vi "Is OceanOptics installed.vi"(8 "Error In":errorcluster) -> (0 "Error Out":errorcluster, 3 "file or folder exists?":bool)   [LabVIEW 2016]
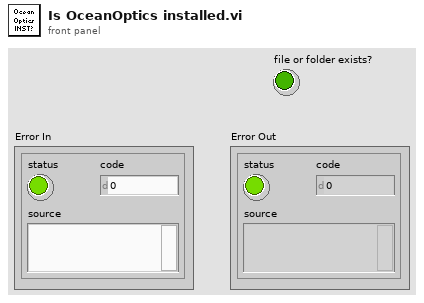
[diagram p1: front panel]
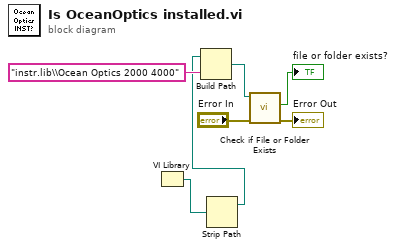
[diagram p0: block diagram]
diagram:
  n1 = VI Library() -> (path=w2:path)
  n2 = Strip Path(path=w2) -> (stripped path=w1:path)  [unwired: 1 out]
  n3 = Build Path(base path=w1, name or relative path="instr.lib\\Ocean Optics 2000 4000") -> (appended path=w6:path)
  n4 = call <vilib>:"Check if File or Folder Exists.vi"("error in (no error)"="Error In", "path"=w6) -> ("error out"=→"Error Out":errorcluster, "file or folder exists?"=→"file or folder exists?":bool)  [unwired: 7 in, 1 out]
